vi "Configure Input RES TRAN MODE.vi"(8 "error in (no error)":errorcluster, 10 "Tran Mode":string(combo)="CONT", 11 "VISA resource name":refnum<visa-resource-name>) -> (0 "error out":errorcluster, 3 "VISA resource name out":refnum<visa-resource-name>)   [LabVIEW 2015, in "IT8900A-E.lvlib"]
doc: "This command selects the operating mode of the transient generator in the following CR mode.\n: CONTinuous transient generator emits a CONTinuous pulse stream after receiving a trigger signal.\n: PULSe transient generator emits a single PULSe after receiving a trigger signal.\n: TOGGle transient generator flips between two values after receiving a trigger signal."
uses:
  <instrlib>/IT8900/IT8900A-E.lvlib
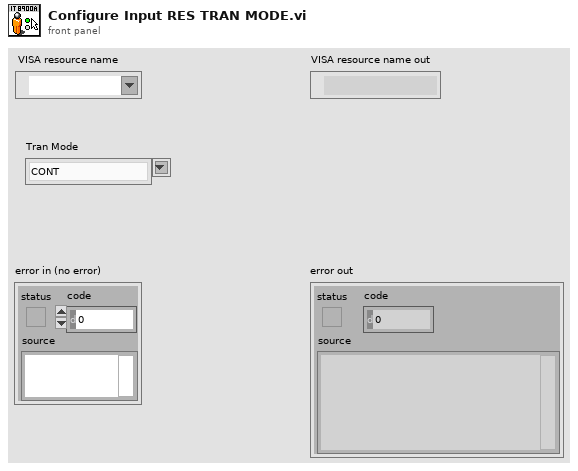
[diagram p1: front panel]
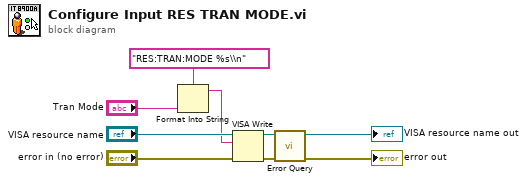
[diagram p0: block diagram]
diagram:
  n1 = Format Into String(format string="RES:TRAN:MODE %s\\n", "Tran Mode") -> (resulting string=w3:string)  [unwired: 2 in, 1 out]
  n2 = VISA Write(VISA resource name="VISA resource name", write buffer=w3, error in (no error)="error in (no error)") -> (VISA resource name out=w6:refnum<visa-resource-name>, error out=w7:errorcluster)  [unwired: 1 out]
  n3 = call <instrlib>:"Error Query.vi"("error in (no error)"=w7, "VISA resource name"=w6) -> ("error out"=→"error out":errorcluster, "VISA resource name out"=→"VISA resource name out":refnum<visa-resource-name>)  [unwired: 6 in, 2 out]
